vi "New Terminal Reference Binding.vi"(9 "Signaling Write? (T)":bool=TRUE, 10 "Ctl Refnum":refnum<vi>) -> (0 "error out":errorcluster, 3 "TerminalReferenceBinding":refnum<class "TerminalReference.lvclass">)   [LabVIEW 2015, in "Transport.lvlib" / "TerminalReference.lvclass"]
doc: "<License>\nCopyright © 2017 Composed Systems, LLC | All rights reserved\nwww.composed.io\n\nAuthor: Ethan Stern <ethan.stern@composed.io>\n\nThis software is provided \"AS IS\" WITHOUT WARRANTIES, either express or implied, AND IS FOR EDUCATIONAL PURPOSES ONLY.\n</License>"
uses:
  TerminalReference.lvclass
  TerminalReference.lvclass/TerminalReference.ctl
  <vilib>/Utility/error.llb/Error Cluster From Error Code.vi
  <vilib>/ErrorRing/Error Ring.xnode
  <vilib>/Utility/Data Type/NI_Data Type.lvlib
panel:
  # "If you don't need Value(Sgnl) writes, use the\nTerminalBinding transport type--it is much faster."
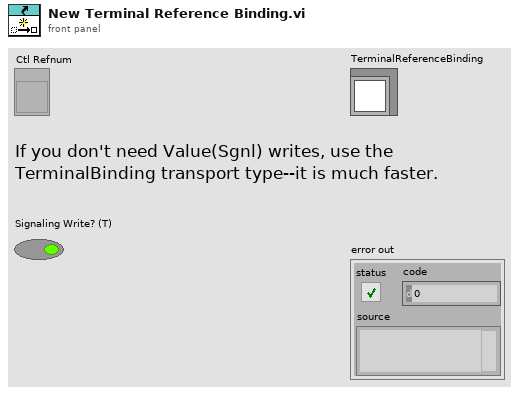
[diagram p1: front panel]
types:
  T1 = typedef "NI_Data Type.lvlib/Data Type.ctl" = enum8{"Invalid Type", "Void", "I8", "I16", "I32", "I64", "U8", "U16", "U32", "U64", "Single Float", "Double Float", "Extended Float", "Single Complex", "Double Complex", "Extended Complex", "Enum U8", "Enum U16", "Enum U32", "Enum U64", "Single Float With Unit", "Double Float With Unit", "Extended Float With Unit", "Single Complex with Unit", "Double Complex with Unit", "Extended Complex with Unit", "Boolean", "String", "Path", "Picture", "Tag", "Array", "Cluster", "Variant", "LV Variant", "Waveform", "Timestamp", "Digital Waveform", "Digital Data", "ExpressData", "Refnum", "External Data", "VI", "Poly VI", "LabVIEW Class Instance", "Fixed Point"}
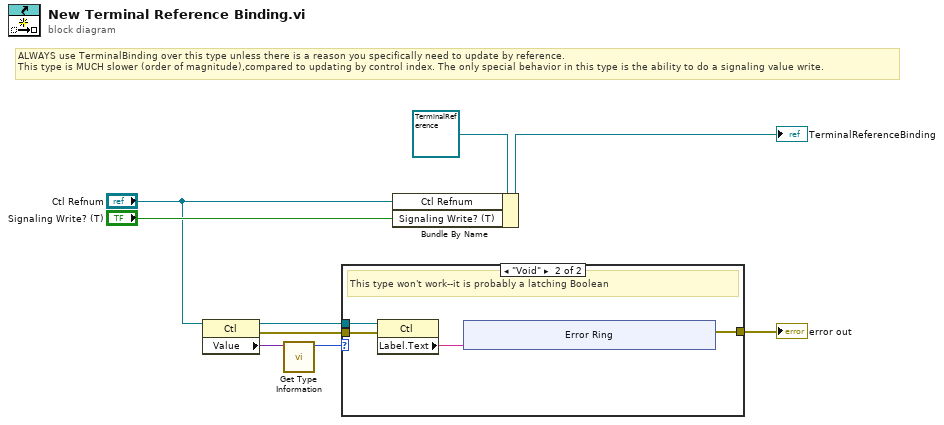
[diagram p0: block diagram]
diagram:
  # "ALWAYS use TerminalBinding over this type unless there is a reason you specifically need to update by reference.\nThis type is MUCH slower (order of magnitude),compared to updating by control index. The only special behavior in this type is the ability to do a signaling value write."
  n1 = property class="Ctl"(reference="Ctl Refnum") -> (reference out=w3:refnum<vi>, error out=w2:errorcluster, "Value"=w6:variant)  [unwired: 1 in]
  n2 = call <vilib>:"Get Type Information.vi"("Variant"=w6) -> ("Type"=w4:T1)  [unwired: 6 in, 4 out]
  n3 = case shown="\"Void\"" w4 {
    tunnel: w3 -> [_ w13]
    tunnel: w2 -> [_ w12]
    tunnel: [_ w10] -> w1
    frame Default {
      # "Valid TerminalReferenceBinding type"
    }
    frame "Void" {
      # "This type won't work--it is probably a latching Boolean"
      n4 = property class="Ctl"(reference=w13, error in=w12) -> ("Label.Text"=w11:string)  [unwired: 2 out]
      n5 = xnode "Error Ring"("parameter 0"=w11) -> ("error out"=w10:errorcluster)
    }
  }
  "error out" <- w1
  n6 = Bundle By Name(cluster=refnum<class "TerminalReference.lvclass"> refnum ("TerminalReference in"), "Ctl Refnum"="Ctl Refnum", "Signaling Write? (T)"="Signaling Write? (T)") -> (→"TerminalReferenceBinding":refnum<class "TerminalReference.lvclass">)
